vi "Get Current Temperature.vi"(8 "error in (no error)":errorcluster, 11 "Simulated Evaporative Cooler":refnum<class "Simulated Evaporative Cooler.lvclass">) -> (0 "error out":errorcluster, 2 "Level":dbl)   [LabVIEW 2025, in "Simulated Evaporative Cooler.lvclass"]
doc: "This VI reads the current indoor air temperature."
uses:
  Simulated Evaporative Cooler.lvclass
  Simulation Data_Global.vi
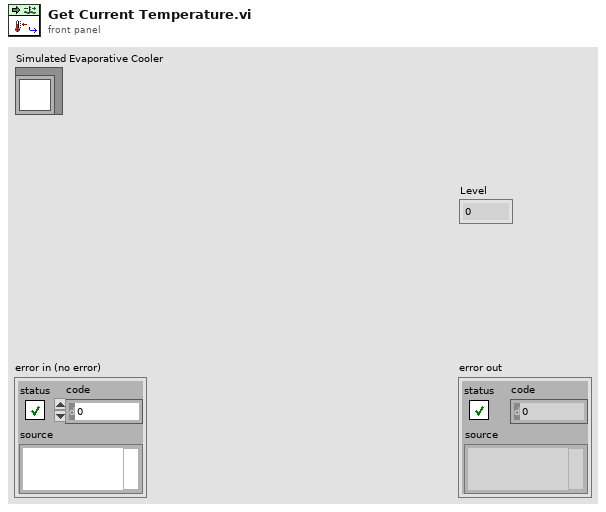
[diagram p1: front panel]
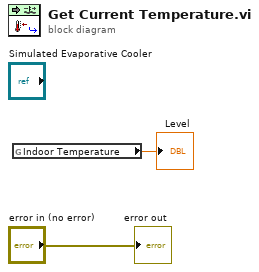
[diagram p0: block diagram]
diagram:
  n1 = global read "Simulation Data_Global.vi" "Indoor Temperature"() -> (→"Level":dbl)
  "error out" <- "error in (no error)"
